vi "CLSUIP_FindCtrlTermOnConPane.vi"(3 "error in (no error)":errorcluster, 4 "Ctl Refnum":refnum<vi>, 5 "ConPane":refnum<vi>) -> (0 "error out":errorcluster, 1 "Terminal Index":i32, 2 "ConPane out":refnum<vi>)   [LabVIEW 2021, in "MemberVICreation.lvlib"]
uses:
  <resource>/Framework/Providers/LVClassLibrary/NewAccessors/MemberVICreation.lvlib
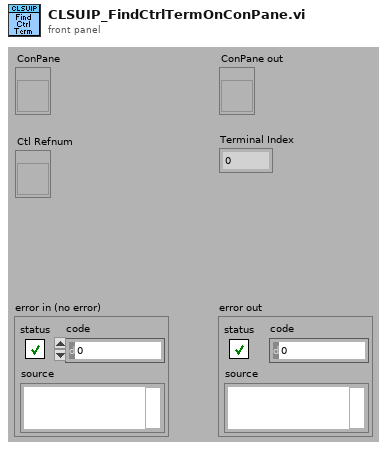
[diagram p1: front panel]
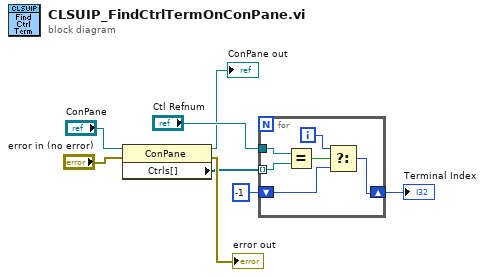
[diagram p0: block diagram]
diagram:
  n1 = property class="ConPane"(reference="ConPane", error in="error in (no error)") -> (reference out=→"ConPane out":refnum<vi>, error out=→"error out":errorcluster, "Ctrls[]"=w3:refnum<vi>[])
  n2 = for {
    tunnel: w3 -> [w13] mode=indexing
    tunnel: "Ctl Refnum" -> [w14]
    shift-right: [w10] -> w6
    shift-left: -1 -> [w9]
    i -> [w11]
    n3 = Equal?(x=w14, y=w13) -> (x = y?=w12:bool)
    n4 = Select(t=w11, s=w12, f=w9) -> (s? t:f=w10:i32)
  }
  "Terminal Index" <- w6
